vi "Simple GPIB.vi"() -> ()   [LabVIEW 2020]
doc: "Demonstrates how to communicate with a GPIB instrument with the GPIB Write and GPIB Read functions."
panel:
  out "Response":string
  in  "GPIB Address":string="1"
  # "Overview: Demonstrates the use of the GPIB functions to communicate to a GPIB instrument.\nRequirements: NI-488.2 Driver\nInstructions:\n1. Ensure the resource specified by the GPIB Address control is properly configured in Measurement & Automation Explorer.\n2. Run the VI.\n3. If your instrument recognizes the \"*IDN?\" command, it should return a Response."
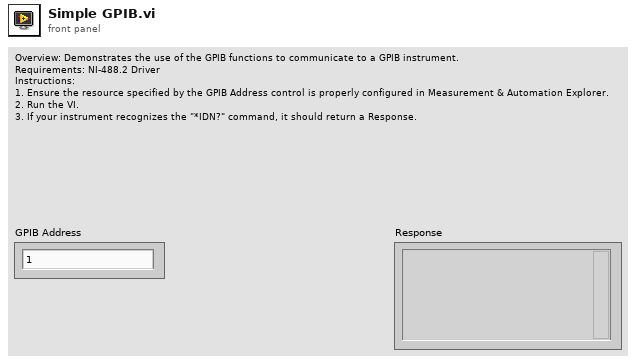
[diagram p1: front panel]
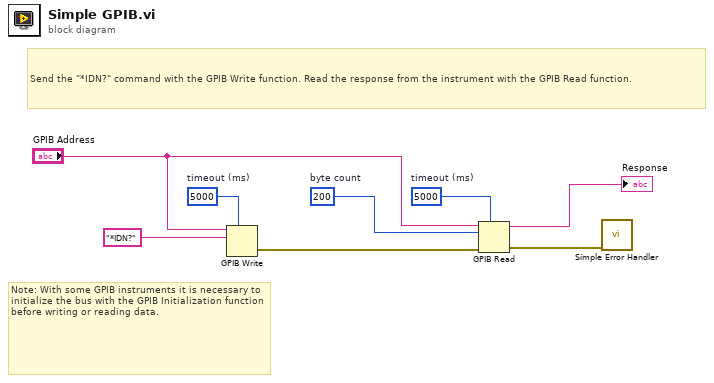
[diagram p0: block diagram]
diagram:
  w1 = 5000  # timeout (ms)
  w4 = 200  # byte count
  w3 = 5000  # timeout (ms)
  # "Note: With some GPIB instruments it is necessary to initialize the bus with the GPIB Initialization function before writing or reading data."
  # "Send the \"*IDN?\" command with the GPIB Write function. Read the response from the instrument with the GPIB Read function."
  n1 = GPIB Write(0:"GPIB Address", 1:"*IDN?" ("Characters to Write"), 4:w3) -> (6:w7:errorcluster)  [unwired: 2 in, 1 out]
  n2 = GPIB Read(0:"GPIB Address", 1:w4, 3:w7, 4:w1) -> (5:→"Response":string, 7:w6:errorcluster)  [unwired: 1 in, 1 out]
  n3 = call <vilib>:"Simple Error Handler.vi"("error in (no error)"=w6) -> ()  [unwired: 4 in, 5 out]
